vi "Execute Measurement.vi"(0 "Measurement Client Wrapper":refnum<class "Measurement Client Wrapper.lvclass">, 11 "error in":errorcluster) -> (4 "Measurement Client Wrapper out":refnum<class "Measurement Client Wrapper.lvclass">, 15 "error out":errorcluster)   [LabVIEW 2020, in "Measurement Client Wrapper.lvclass"]
uses:
  Measurement Client Wrapper.lvclass
  Measurement Client Wrapper.lvclass/Measurement Client Wrapper.ctl
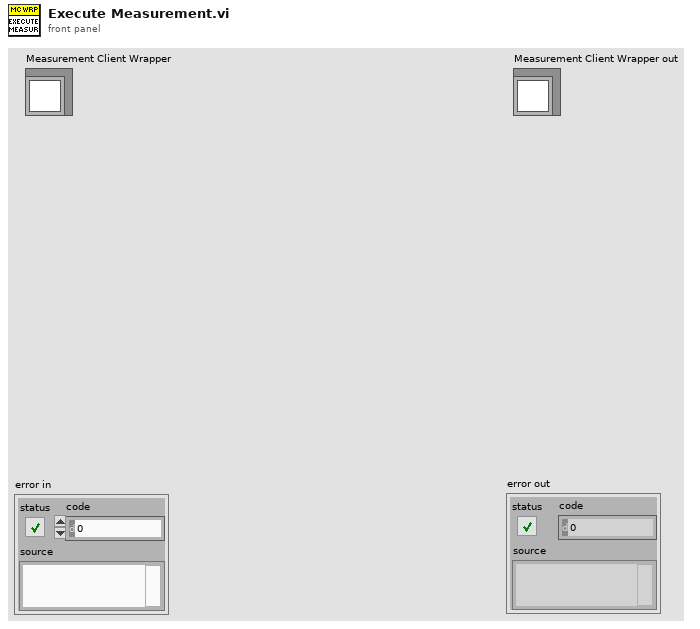
[diagram p1: front panel]
types:
  T1 = typedef "Measurement Client Wrapper.lvclass/MeasurementConfigurationParameters.ctl" = cluster{"protobuf_id":u32, "type":T2, "name":string, "repeated":bool}
  T2 = typedef "Measurement_client-release.lvlib/google_protobuf_Field_Kind.ctl" = enum32{"TYPE_UNKNOWN", "TYPE_DOUBLE", "TYPE_FLOAT", "TYPE_INT64", "TYPE_UINT64", "TYPE_INT32", "TYPE_FIXED64", "TYPE_FIXED32", "TYPE_BOOL", "TYPE_STRING", "TYPE_GROUP", "TYPE_MESSAGE", "TYPE_BYTES", "TYPE_UINT32", "TYPE_ENUM", "TYPE_SFIXED32", "TYPE_SFIXED64", "TYPE_SINT32", "TYPE_SINT64"}
  T3 = typedef "Measurement Client Wrapper.lvclass/MeasurementOutputParameters.ctl" = cluster{"protobuf_id":u32, "type":T2, "name":string, "repeated":bool}
  T4 = typedef "Measurement Client Wrapper.lvclass/Control UI MetaData.ctl" = cluster{"Name":string, "Parent":string, "LabVIEW DataType":T5, "Measurement DataType":T2, "Value":variant, "1D Array?":bool}
  T5 = typedef "NI_Data Type.lvlib/Data Type.ctl" = enum8{"Invalid Type", "Void", "I8", "I16", "I32", "I64", "U8", "U16", "U32", "U64", "Single Float", "Double Float", "Extended Float", "Single Complex", "Double Complex", "Extended Complex", "Enum U8", "Enum U16", "Enum U32", "Enum U64", "Single Float With Unit", "Double Float With Unit", "Extended Float With Unit", "Single Complex with Unit", "Double Complex with Unit", "Extended Complex with Unit", "Boolean", "String", "Path", "Picture", "Tag", "Array", "Cluster", "Variant", "LV Variant", "Waveform", "Timestamp", "Digital Waveform", "Digital Data", "ExpressData", "Refnum", "External Data", "VI", "Poly VI", "LabVIEW Class Instance", "Fixed Point", "Set Collection", "Map Collection"}
  T6 = cluster{"type":T2, "repeated":bool, "Value":variant}
  T7 = cluster{"Measurement DataType":T2, "Array Dimension":bool, "Data":variant}[]
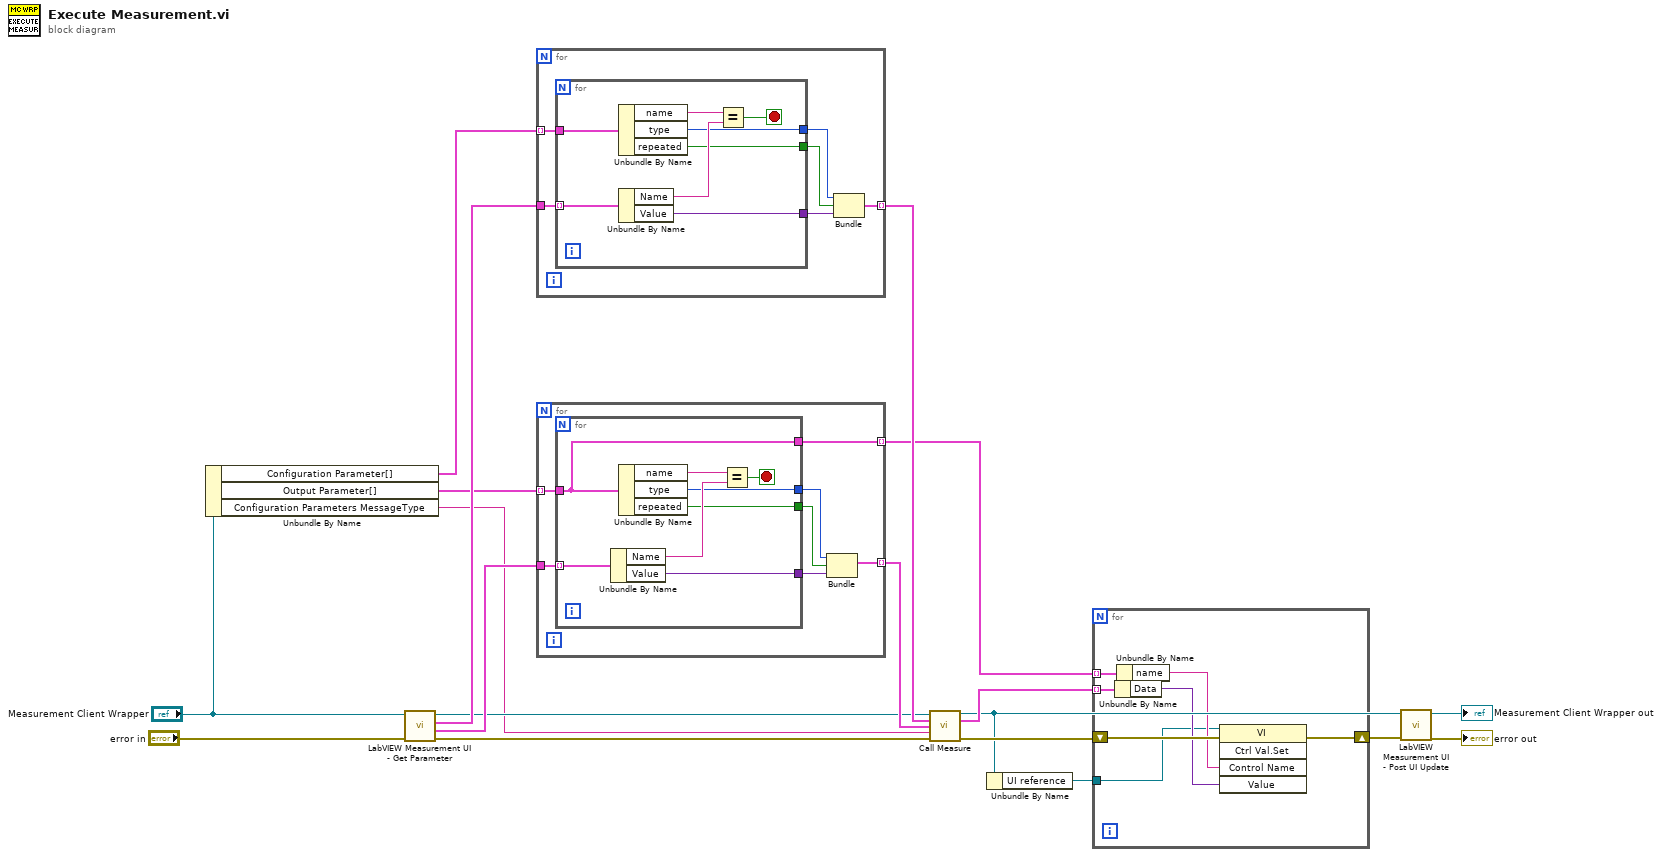
[diagram p0: block diagram]
diagram:
  n1 = Unbundle By Name("Measurement Client Wrapper") -> ("Configuration Parameter[]"=w3:T1[], "Output Parameter[]"=w8:T3[], "Configuration Parameters MessageType"=w1:string)
  n2 = call "LabVIEW Measurement UI - Get Parameter.vi"("error in"="error in", "Measurement Client Wrapper in"="Measurement Client Wrapper") -> ("error out"=w18:errorcluster, "UI Indicator Details[]"=w15:T4[], "UI Control Details[]"=w17:T4[], "Measurement Client Wrapper"=w10:refnum<class "Measurement Client Wrapper.lvclass">)  [unwired: 6 in]
  n3 = for {
    tunnel: w3 -> [w24] mode=indexing
    tunnel: w17 -> [w25]
    tunnel: [w21] -> w16 mode=indexing
    n4 = for {
      tunnel: w25 -> [w33] mode=indexing
      tunnel: w24 -> [w30]
      tunnel: [w29] -> w22
      tunnel: [w28] -> w23
      tunnel: [w27] -> w20
      stop <- w26 stop-if-true
      n5 = Unbundle By Name(w30) -> ("name"=w31:string, "type"=w28:T2, "repeated"=w27:bool)
      n6 = Unbundle By Name(w33) -> ("Name"=w32:string, "Value"=w29:variant)
      n7 = Equal?(x=w31, y=w32) -> (x = y?=w26:bool)
    }
    n8 = Bundle("type"=w23, "repeated"=w20, "Value"=w22) -> (w21:T6)  [unwired: 1 in]
  }
  n9 = for {
    tunnel: w8 -> [w39] mode=indexing
    tunnel: w15 -> [w40]
    tunnel: [w36] -> w14 mode=indexing
    tunnel: [w35] -> w12 mode=indexing
    n10 = for {
      tunnel: w40 -> [w48] mode=indexing
      tunnel: w39 -> [w44]
      tunnel: [w44] -> w35
      tunnel: [w43] -> w37
      tunnel: [w42] -> w38
      tunnel: [w41] -> w34
      stop <- w46 stop-if-true
      n11 = Unbundle By Name(w48) -> ("Name"=w47:string, "Value"=w43:variant)
      n12 = Unbundle By Name(w44) -> ("name"=w45:string, "type"=w42:T2, "repeated"=w41:bool)
      n13 = Equal?(x=w45, y=w47) -> (x = y?=w46:bool)
    }
    n14 = Bundle("type"=w38, "repeated"=w34, "Value"=w37) -> (w36:T6)  [unwired: 1 in]
  }
  n15 = call "Call Measure.vi"("Measurement Client Wrapper in"=w10, "Config Data"=w16, "Expected Output Format"=w14, "ConfigurationParametersMessagetype"=w1, "error in (no error)"=w18) -> ("Measurement Client Wrapper out"=w6:refnum<class "Measurement Client Wrapper.lvclass">, "Output Data"=w11:T7, "error out"=w13:errorcluster)  [unwired: 8 in]
  n16 = Unbundle By Name(w6) -> ("UI reference"=w9:refnum<vi>)
  n17 = for {
    shift-right: [w54] -> w7
    shift-left: w13 -> [w55]
    tunnel: w12 -> [w52] mode=indexing
    tunnel: w11 -> [w51] mode=indexing
    tunnel: w9 -> [w49]
    n18 = Unbundle By Name(w51) -> ("Data"=w50:variant)
    n19 = Unbundle By Name(w52) -> ("name"=w53:string)
    n20 = invoke class="VI" method="Ctrl Val.Set"(reference=w49, error in=w55, "Control Name"=w53, "Value"=w50) -> (error out=w54:errorcluster)  [unwired: 1 in, 4 out]
  }
  n21 = call "LabVIEW Measurement UI - Post UI Update.vi"("error in"=w7, "Measurement Client Wrapper in"=w6) -> ("error out"=→"error out":errorcluster, "Measurement Client Wrapper"=→"Measurement Client Wrapper out":refnum<class "Measurement Client Wrapper.lvclass">)  [unwired: 8 in]
